vi "TDMS Concatenate Files.vi"(6 "post defrag? (F)":bool, 8 "error in":errorcluster, 9 "Operation Dest (1: open or create)":T1(ring)=enum."open or create", 10 "Source files":path[](array[path]), 11 "Destination file":path) -> (0 "error out":errorcluster, 2 "Source files out":path[](array[path]), 3 "Destination file out":path)   [LabVIEW 2011]
doc: "Concatenates several tdms files to one new file.\nIf the same channel is present in several source files, the data is appended in the order of the files listed. When a propery exists in more than one source file, the one from the last source file is copied.\n\nIf \"post defrag\"=true the destination file will be defraged after concatenation.\nIf \"error in\" has error the function does nothing and outputs empty values for \"Destination file out\" and \"Source files out\"!"
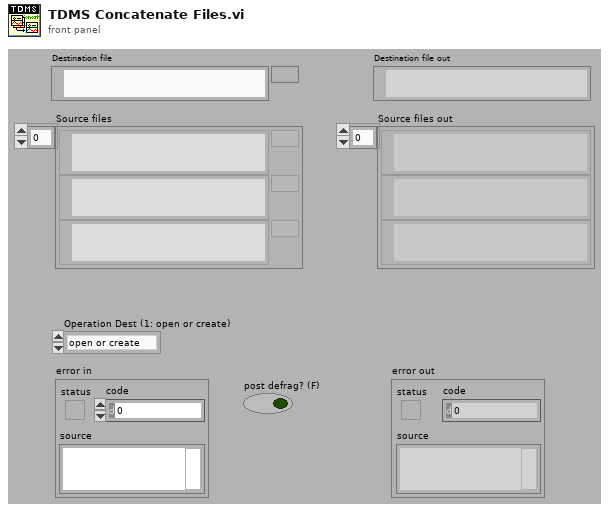
[diagram p1: front panel]
types:
  T1 = enum16{"open", "open or create", "create or replace", "create", "open (read-only)"}
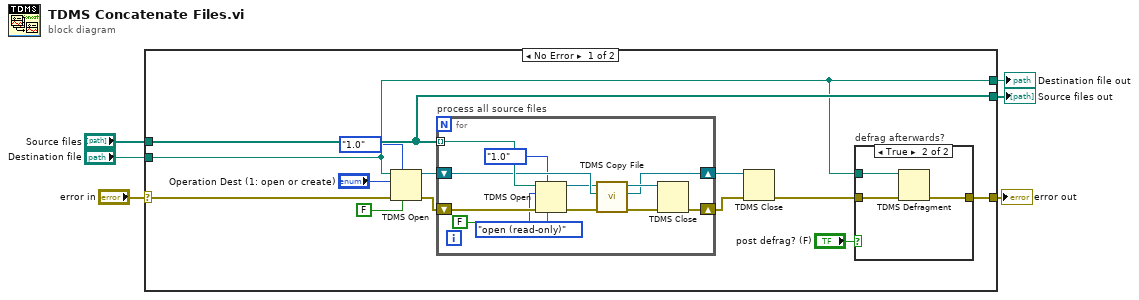
[diagram p0: block diagram]
diagram:
  n1 = case shown="No Error" "error in" {
    selector: "error in" -> [w11 w36]
    tunnel: [w13 w36] -> w6
    tunnel: "Destination file" -> [w9 _]
    tunnel: "Source files" -> [w10 _]
    tunnel: [w10 _] -> w2
    tunnel: [w9 _] -> w1
    frame No Error {
      n2 = TDMS Open(6:FALSE ("disable buffering (T)"), 7:enum16{"1.0", "2.0"}."1.0" ("file format version (2.0)"), 8:w11, 10:"Operation Dest (1: open or create)", 11:w9) -> (0:w19:errorcluster, 3:w18:refnum<k34>)  [unwired: 1 in]
      n3 = for "process all source files" {
        shift-right: [w35] -> w16
        shift-left: w19 -> [w34]
        shift-right: [w28] -> w17
        shift-left: w18 -> [w31]
        tunnel: w10 -> [w33] mode=indexing
        n4 = TDMS Open(6:FALSE ("disable buffering (T)"), 7:enum16{"1.0", "2.0"}."1.0" ("file format version (2.0)"), 8:w34, 10:T1."open (read-only)" ("Operation (0:Öffnen)"), 11:w33) -> (0:w26:errorcluster, 3:w30:refnum<k34>)  [unwired: 1 in]
        n5 = call "TDMS Copy File.vi"("error in"=w26, "tdms dest in"=w31, "tdms source in"=w30) -> ("error out"=w27:errorcluster, "tdms dest out"=w28:refnum<k34>, "tdms source out"=w29:refnum<k34>)  [unwired: 1 in, 5 out]
        n6 = TDMS Close(8:w27, 11:w29) -> (0:w35:errorcluster)  [unwired: 1 out]
      }
      n7 = TDMS Close(8:w16, 11:w17) -> (0:w14:errorcluster)  [unwired: 1 out]
      n8 = case "defrag afterwards?" shown="True" "post defrag? (F)" {
        tunnel: w14 -> [w20 w23]
        tunnel: [w20 w22] -> w13
        tunnel: w9 -> [_ w21]
        frame False {
          # "do nothing"
        }
        frame True {
          n9 = TDMS Defragment(4:w23, 7:w21) -> (0:w22:errorcluster)
        }
      }
    }
    frame Error {
      # "check if empty for\nerror is OK?"
    }
  }
  "error out" <- w6
  "Source files out" <- w2
  "Destination file out" <- w1
